vi "Loop Control.vi"(8 "error in (no error)":errorcluster, 9 "Loop Type":string, 10 "Controller #":string, 11 "Port In":T1) -> (0 "error out":errorcluster, 3 "Port Out":T1)   [LabVIEW 2021]
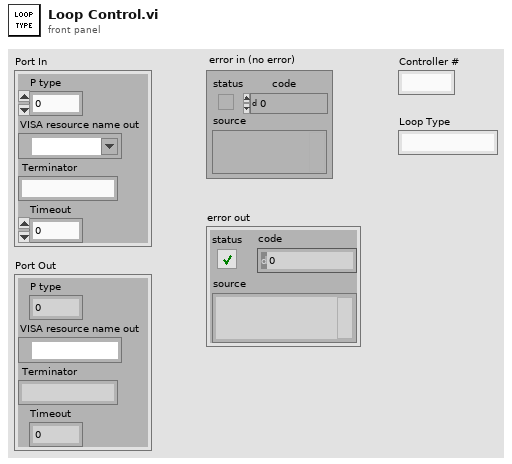
[diagram p1: front panel]
types:
  T1 = cluster{"P type":u16, "VISA resource name out":refnum<visa-resource-name>, " Terminator":string, "Timeout":i32}
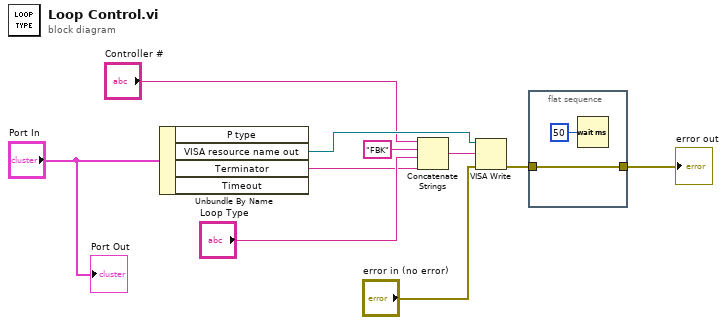
[diagram p0: block diagram]
diagram:
  n1 = Unbundle By Name("Port In") -> ("VISA resource name out"=w7:refnum<visa-resource-name>, "Terminator"=w3:string)  [unwired: 2 out]
  n2 = Concatenate Strings("Controller #", "FBK" ("string"), "Loop Type", w3) -> (w9:string)
  n3 = VISA Write(VISA resource name=w7, write buffer=w9, error in (no error)="error in (no error)") -> (error out=w2:errorcluster)  [unwired: 2 out]
  n4 = flat-sequence {
    tunnel: [w12] -> w1
    tunnel: w2 -> [w12]
    frame #0 {
      n5 = Wait (ms)(milliseconds to wait=u32 50) -> ()  [unwired: 1 out]
    }
  }
  "error out" <- w1
  "Port Out" <- "Port In"
